vi "PH_Sixpack.Init.vi"(0 "i ref in":refnum<vi>, 5 "error in":errorcluster) -> (14 "i ref out":refnum<vi>, 18 "Device Error out":errorcluster, 19 "error out":errorcluster)   [LabVIEW 2014, in "PH_Sixpack.lvlib"]
doc: "This VI passes the addressing information in the instrument decriptor to the Instr Open VI and returns the instrument ID. You can optionally reset the instrument by setting the front panel reset control. You must run this VI before using any of the instrument driver VIs for this instrument."
uses:
  PH_Sixpack.lvlib
  instr.lib/Sixpack/Sixpack - Driver.lvlib
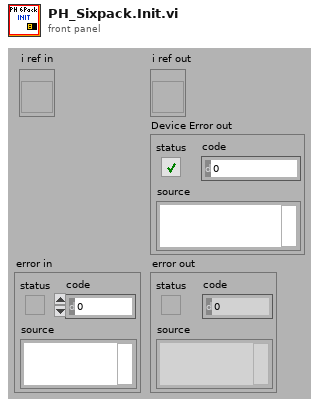
[diagram p1: front panel]
types:
  T1 = typedef "PH_Sixpack.lvlib/PH_Sixpack.i attribute.ctl" = cluster{"Information":cluster{"SixPack ID(0)":u16, "BaudRate(19200)":u16, "COM Port":enum32{"COM1", "COM2", "COM3", "COM4", "COM5", "COM6", "COM7", "COM8", "COM9"}, "HANDLE":i32}, "Serial Number":dbl, "Firmwareversion":dbl, "Axes":T2[], "Status":T14, "Axis to do a RefSearch":i32, "GUI Refs":cluster{"Information":refnum<vi>, "Serial Number":refnum<vi>, "Firmwareversion":refnum<vi>, "Status":refnum<vi>, "Axis to do a RefSearch":refnum<vi>, "Axes Configuration (Sixpack)":refnum<vi>, "Inputs":refnum<vi>, "PeriodicInterval [ms]":refnum<vi>}, "Constructor finished":bool, "Ignore Error":bool}
  T2 = typedef "PH_Sixpack.lvlib/PH_Sixpack.Axis Cluster.ctl" = cluster{"Config":T3, "To set?":cluster{"VmaxAmax":bool, "I max":bool, "VStartVminDivi":bool, "Ref Search Parameter":bool, "Stopswitch Limits":bool, "Axis Parameter":bool, "I Control":bool}}
  T3 = typedef "PH_Sixpack.lvlib/PH_Sixpack.Axis Configuration.ctl" = cluster{"VmaxAmax":T4, "I max (50%)":T5, "VStartVminDivi":T6, "Ref Search Parameter":T7, "Stopswitch Limits":T8, "Axis Parameter":T9, "I Control":T12}
  T4 = typedef "Sixpack - Driver.lvlib/VmaxAmax.ctl" = cluster{"VMax(511)":u16, "AMax(128)":u16}
  T5 = typedef "Sixpack - Driver.lvlib/PeakCurrent.ctl" = dbl
  T6 = typedef "Sixpack - Driver.lvlib/VStartVmin.ctl" = cluster{"VStart(5)":u16, "Vmin(4)":u16, "Div i (2)":enum8{"0", "1", "2", "3"}}
  T7 = typedef "Sixpack - Driver.lvlib/Ref Search Parameter.ctl" = cluster{"VRefMax(100)":u16, "DebouncingTime (22ms)":u8}
  T8 = typedef "Sixpack - Driver.lvlib/Stopswitch Limits.ctl" = cluster{"MinLeft(0)":u16, "MaxRight(1023)":u16}
  T9 = typedef "Sixpack - Driver.lvlib/Motor Parameter.ctl" = cluster{"Poslimit (6400)":u32, "P5 Bits":T10, "P6 Bits":T11}
  T10 = typedef "Sixpack - Driver.lvlib/MotorParameter_P5.ctl" = cluster{"MT_PI":bool, "MT_ROTARY":bool, "MT_AUTONULLCMD":bool, "MT_TESTNULL":bool, "MT_NULLLEFT":bool, "MT_NULLCENTRE":bool, "MT_STOPNULL":bool, "MT_FILTERSWITCH":bool}
  T11 = typedef "Sixpack - Driver.lvlib/MotorParameter_P6.ctl" = cluster{"MT_OPTIMIZEWAY":bool, "MT_FASTREF":bool, "MT_MECHREF":bool, "MT_DELAYTESTNULL":bool, "MT_STOPSOFT":bool, "MT_STOPNOREF":bool, "MT_NULLPOSITIVE":bool, "MUT_STOPFULSTEPS":bool}
  T12 = typedef "Sixpack - Driver.lvlib/Current Control.ctl" = cluster{"PowerDownDelay (500)":u16, "PowerDown (0%)":T13, "Standing (50%)":T13, "Running (75%)":T13, "Accelerating (100%)":T13}
  T13 = typedef "Sixpack - Driver.lvlib/Current.ctl" = enum8{"100%", "75%", "50%", "38%", "25%", "19%", "13%", "9%", "0%"}
  T14 = typedef "PH_Sixpack.lvlib/PH_Sixpack.Status.ctl" = enum32{"None", "Init", "Configure", "configured", "Close", "closed"}
  T15 = enum32{"COM1", "COM2", "COM3", "COM4", "COM5", "COM6", "COM7", "COM8", "COM9"}
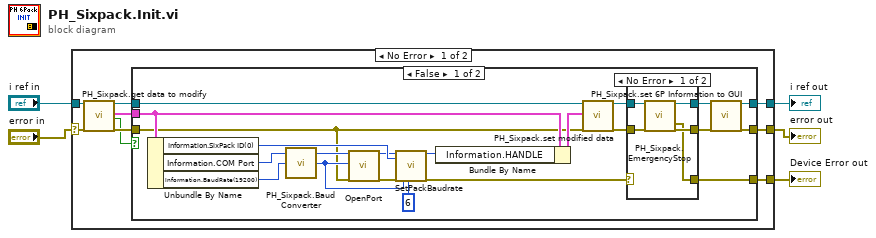
[diagram p0: block diagram]
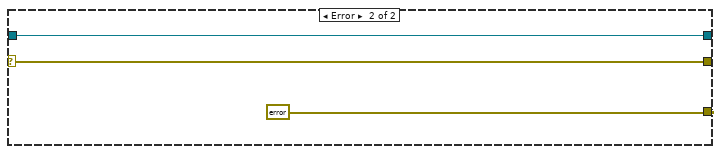
[diagram p4: hidden frame]
diagram:
  n1 = case shown="No Error" "error in" {
    selector: "error in" -> [w8 w47]
    tunnel: "i ref in" -> [w14 w48]
    tunnel: [w13 w47] -> w4
    tunnel: [w12 w48] -> w3
    tunnel: [w6 errorcluster {"status"=FALSE, "code"=0, "source"=""} ("error out")] -> w1
    frame No Error {
      n2 = call "PH_Sixpack.get data to modify.vi"("i ref in"=w14, "error in (no error)"=w8) -> ("i ref out"=w11:refnum<vi>, "i attribute"=w9:T1, "timed out"=w7:bool, "error out"=w10:errorcluster)  [unwired: 14 in]
      n3 = case shown="False" w7 {
        tunnel: [w21 w44] -> w13
        tunnel: [w22 w45] -> w12
        tunnel: w11 -> [w34 w45]
        tunnel: w10 -> [w23 w44]
        tunnel: w9 -> [w24 _]
        tunnel: [w16 errorcluster {"status"=FALSE, "code"=0, "source"=""} ("error out")] -> w6
        frame False {
          n4 = Unbundle By Name(w24) -> ("Information.SixPack ID(0)"=w32:u16, "Information.COM Port"=w25:T15, "Information.BaudRate(19200)"=w33:u16)
          n5 = call "PH_Sixpack.Baud Converter.vi"("BaudRate(19200)"=w33) -> ("BaudRate (19200)"=w26:enum32{"9600", "19200", "38400", "57600"})
          n6 = call "OpenPort.vi"("COM Port (COM1)"=w25, "BaudRate (19200)"=w26, "error in (no error)"=w23) -> ("handle"=w30:i32, "error out"=w27:errorcluster)  [unwired: 15 in]
          n7 = call "SetPackBaudrate.vi"("handle in"=w30, "UnitAddress(0)"=w32, "error in"=w27, "BaudRate (19200)"=w26, "Delay(6)"=u16 6 ("Delay")) -> ("handle out"=w28:i32, "error out"=w15:errorcluster)  [unwired: 13 in]
          n8 = Bundle By Name(cluster=w24, "Information.HANDLE"=w28) -> (w31:T1)
          n9 = call "PH_Sixpack.set modified data.vi"("i ref in"=w34, "i attribute"=w31, "error in (no error)"=w23) -> ("i ref out"=w20:refnum<vi>, "error out"=w18:errorcluster)  [unwired: 15 in]
          n10 = case shown="No Error" w15 {
            selector: w15 -> [_ w42]
            tunnel: w20 -> [w39 w40]
            tunnel: [w38 w40] -> w19
            tunnel: w18 -> [w37 w41]
            tunnel: [w36 w41] -> w17
            tunnel: [w35 w42] -> w16
            frame No Error {
              n11 = call "PH_Sixpack.EmergencyStop.vi"("i ref in"=w39, "error in"=w37) -> ("i ref out"=w38:refnum<vi>, "Device Error out"=w35:errorcluster, "error out"=w36:errorcluster)  [unwired: 15 in]
            }
            frame Error {
            }
          }
          n12 = call "PH_Sixpack.set 6P Information to GUI.vi"("VI in"=w19, "error in (no error)"=w17) -> ("VI out"=w22:refnum<vi>, "error out"=w21:errorcluster)  [unwired: 16 in]
        }
        frame True {
        }
      }
    }
    frame Error {
    }
  }
  "error out" <- w4
  "i ref out" <- w3
  "Device Error out" <- w1
